vi "Parse maps.vi"(11 "string in":string) -> (2 "map":T1, 3 "string out":string)   [LabVIEW 2023, in "d5.lvlib"]
uses:
  d5.lvlib
  74905e41-61e0-44e3-8266-22c235a8375f.vi
  <vilib>/regexp/Match Regular Expression.xnode
  <vilib>/Comparison/Less/Less Functor/Less Functor.lvclass
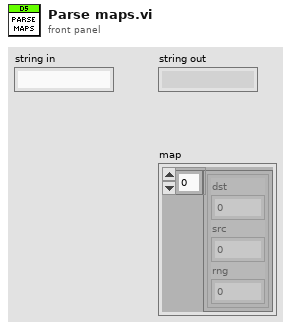
[diagram p1: front panel]
types:
  T1 = cluster{cluster{"dst":i64, "src":i64, "rng":i64}[]}
  T2 = cluster{"default value 1":i64, "default value 1":i64, "default value 1":i64}
  T3 = cluster{"default value 1":i64, "default value 1":i64, "default value 1":i64}[]
  T4 = cluster{cluster{"default value 1":i64, "default value 1":i64, "default value 1":i64}[]}
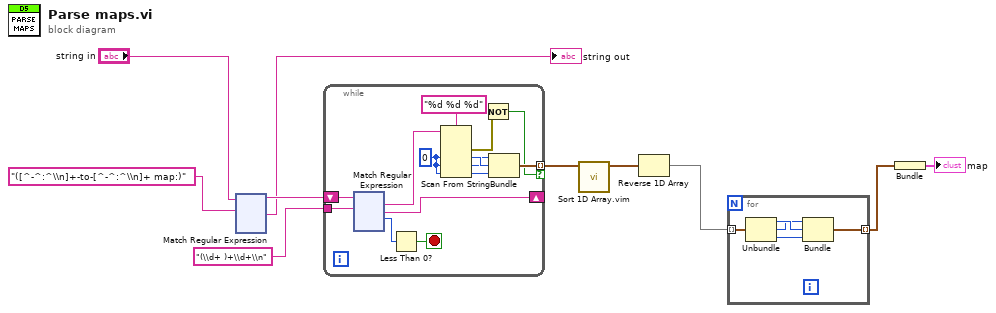
[diagram p0: block diagram]
diagram:
  n1 = xnode "Match Regular Expression"("input string"="string in", "regular expression"="([^-^:^\\n]+-to-[^-^:^\\n]+ map:)") -> ("before match"=w10:string, "after match"=→"string out":string)  [unwired: 4 in, 3 out]
  n2 = while {
    tunnel: "(\\d+ )+\\d+\\n" ("regular expression") -> [w23]
    shift-right: [w22] -> _
    shift-left: w10 -> [w24]
    tunnel: [w16] -> w4 mode=indexing if=w14
    stop <- w20 stop-if-true
    w13 = i64 0 ("default value 1")
    n3 = xnode "Match Regular Expression"("input string"=w24, "regular expression"=w23) -> ("whole match"=w19:string, "after match"=w22:string, "offset past match"=w21:i32)  [unwired: 4 in, 2 out]
    n4 = Less Than 0?(x=w21) -> (x < 0?=w20:bool)
    n5 = Scan From String(format string="%d %d %d", input string=w19, default 1=w13, default 2=w13, default 3=w13) -> (error out=w15:errorcluster, output 1=w12:i64, output 2=w11:i64, output 3=w17:i64)  [unwired: 2 in, 2 out]
    n6 = Not(x=w15) -> (.not. x?=w14:bool)
    n7 = Bundle("default value 1"=w11, "default value 1"=w12, "default value 1"=w17) -> (w16:T2)  [unwired: 1 in]
  }
  n8 = call "Sort 1D Array.vim"("unsorted array"=w4) -> ("sorted array"=w3:T3)  [unwired: 10 in]
  n9 = Reverse 1D Array(array=w3) -> (reversed array=w2:T3)
  n10 = for {
    tunnel: w2 -> [w146] mode=indexing
    tunnel: [w142] -> w1 mode=indexing
    n11 = Unbundle(w146) -> ("default value 1"=w144:i64, "default value 1"=w143:i64, "default value 1"=w145:i64)
    n12 = Bundle("default value 1"=w143, "default value 1"=w144, "default value 1"=w145) -> (w142:T2)  [unwired: 1 in]
  }
  n13 = Bundle(w1) -> (→"map":T4)  [unwired: 1 in]
